vi "DAQPhysicalNameToCardChannelNumbers.vi"(3 "NI Physical Channel":string="DAQ1/ai6") -> (0 "Channel #":string, 1 "Card #":string)   [LabVIEW 2014]
doc: "VI that grabs the DAQ card/channel# from the PXI physical address, and outputs them as strings for use in tagging via 'for' loops. Note that these are hard-coded for the 'DAQs' (2.5MHz cards)."
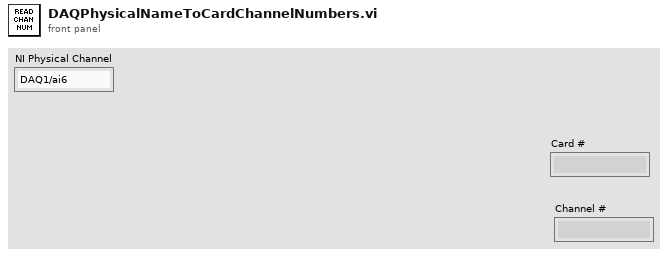
[diagram p1: front panel]
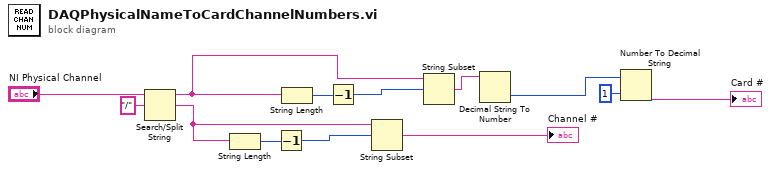
[diagram p0: block diagram]
diagram:
  n1 = Search/Split String(string="NI Physical Channel", search string/char (-)="/") -> (substring before match=w11:string, match + rest of string=w5:string)  [unwired: 1 in, 1 out]
  n2 = String Length(string=w5) -> (length=w7:i32)
  n3 = Decrement(x=w7) -> (x-1=w8:i32)
  n4 = String Length(string=w11) -> (length=w10:i32)
  n5 = Decrement(x=w10) -> (x-1=w9:i32)
  n6 = String Subset(string=w5, offset (0)=w8) -> (substring=→"Channel #":string)  [unwired: 1 in]
  n7 = String Subset(string=w11, offset (0)=w9) -> (substring=w4:string)  [unwired: 1 in]
  n8 = Decimal String To Number(string=w4) -> (number=w1:i32)  [unwired: 2 in, 1 out]
  n9 = Number To Decimal String(number=w1, width (-)=i16 1) -> (decimal integer string=→"Card #":string)
